vi "FestoCPX.Station.ProdSuctionGripper.SetAll.vi"(8 "error in":errorcluster, 10 "Position":T1) -> (0 "error out":errorcluster)   [LabVIEW 2016]
uses:
  Station/Station.ValvePosition.ctl
  FestoCPX.DO.Signal.ctl
  Station/Station.ProductSuctionGripper.Type.ctl
  FestoCPX.DO.Data.States.Set.vi
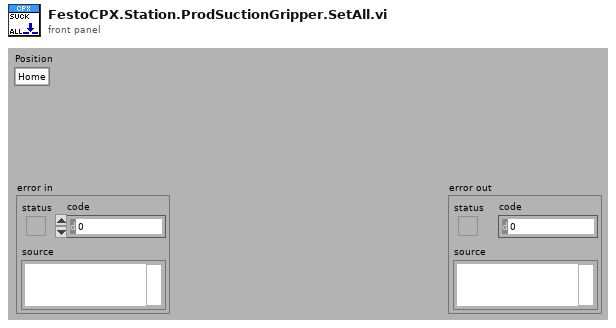
[diagram p1: front panel]
types:
  T1 = typedef "Station.ValvePosition.ctl" = enum16{"Home", "Work"}
  T2 = typedef "FestoCPX.DO.Signal.ctl" = enum16{"Safety Reset", "Air Main Valve", "Door Lock", "Button LED Start", "Button LED Stop", "Button LED Control", "Traffic LED Red", "Traffic LED Orange", "Traffic LED Green", "Horn", "Laser Interlock", "Laser Trigger", "Laser Fume Extractor", "Product Suction Gripper Slot 1 A", "Product Suction Gripper Slot 1 B", "Product Suction Gripper Slot 2 A", "Product Suction Gripper Slot 2 B", "Product Suction Gripper Slot 3 A", "Product Suction Gripper Slot 3 B", "Product Suction Gripper Slot 4 A", "Product Suction Gripper Slot 4 B", "Product Suction Gripper Final A", "Product Suction Gripper Final B", "Lamp", "Q1 Product Move Work", "Q1 Product Move Home", "Q2 Table Turn Work", "Q2 Table Turn Home", "Q3 Product Lift A", "Q3 Product Lift B", "Q4 Product Arm OK", "Q4 Product Arm NOK", "Q5 Product Arm Work", "Q6 Product BlowOut A", "Q6 Product BlowOut B"}
  T3 = typedef "Station.ProductSuctionGripper.Type.ctl" = enum8{"Final A", "Final B", "Slot 1 A", "Slot 1 B", "Slot 2 A", "Slot 2 B", "Slot 3 A", "Slot 3 B", "Slot 4 A", "Slot 4 B"}
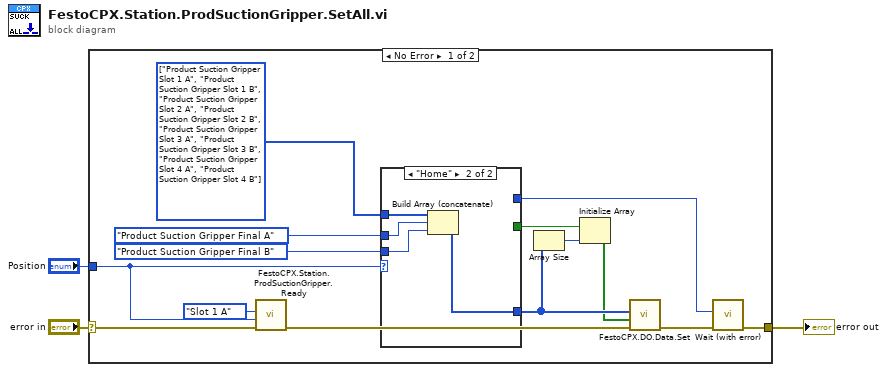
[diagram p0: block diagram]
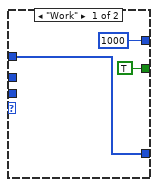
[diagram p2: hidden frame]
diagram:
  n1 = case shown="No Error" "error in" {
    selector: "error in" -> [w16 w25]
    tunnel: [w5 w25] -> w3
    tunnel: "Position" -> [w13 _]
    frame No Error {
      w10 = T2[] [enum."Product Suction Gripper Slot 1 A", enum."Product Suction Gripper Slot 1 B", enum."Product Suction Gripper Slot 2 A", enum."Product Suction Gripper Slot 2 B", enum."Product Suction Gripper Slot 3 A", enum."Product Suction Gripper Slot 3 B", enum."Product Suction Gripper Slot 4 A", enum."Product Suction Gripper Slot 4 B"] items=["Safety Reset", "Air Main Valve", "Door Lock", "Button LED Start", "Button LED Stop", "Button LED Control", "Traffic LED Red", "Traffic LED Orange", "Traffic LED Green", "Horn", "Laser Interlock", "Laser Trigger", "Laser Fume Extractor", "Product Suction Gripper Slot 1 A", "Product Suction Gripper Slot 1 B", "Product Suction Gripper Slot 2 A", "Product Suction Gripper Slot 2 B", "Product Suction Gripper Slot 3 A", "Product Suction Gripper Slot 3 B", "Product Suction Gripper Slot 4 A", "Product Suction Gripper Slot 4 B", "Product Suction Gripper Final A", "Product Suction Gripper Final B", "Lamp", "Q1 Product Move Work", "Q1 Product Move Home", "Q2 Table Turn Work", "Q2 Table Turn Home", "Q3 Product Lift A", "Q3 Product Lift B", "Q4 Product Arm OK", "Q4 Product Arm NOK", "Q5 Product Arm Work", "Q6 Product BlowOut A", "Q6 Product BlowOut B"] ("CPX.DO")
      n2 = call "FestoCPX.Station.ProdSuctionGripper.Ready.vi"("error in"=w16, "Position"=w13, "Type"=Station.ProductSuctionGripper.Type."Slot 1 A") -> ("error out"=w15:errorcluster)  [unwired: 7 in, 1 out]
      n3 = case shown="\"Home\"" w13 {
        tunnel: w10 -> [w20 w24]
        tunnel: FestoCPX.DO.Signal."Product Suction Gripper Final A" ("CPX.DO") -> [_ w23]
        tunnel: FestoCPX.DO.Signal."Product Suction Gripper Final B" ("CPX.DO") -> [_ w22]
        tunnel: [w20 w21] -> w9
        tunnel: [TRUE _] -> w7
        tunnel: [u32 1000 ("milliseconds to wait") _] -> w4
        frame "Work" {
        }
        frame "Home" {
          n4 = Build Array (concatenate)(w24, w23, w22) -> (w21:T2[])
        }
      }
      n5 = Array Size(array=w9) -> (size(s)=w8:i32)
      n6 = Initialize Array(w7, w8) -> (w6:bool[])
      n7 = call-poly "FestoCPX.DO.Data.Set.vi"("error in (no error)"=w15, "State"=w6, "CPX.DO"=w9) -> ("error out"=w17:errorcluster)  [unwired: 8 in]
      n8 = call "Wait (with error).vi"("error in (no error)"=w17, "milliseconds to wait"=w4) -> ("error out"=w5:errorcluster)  [unwired: 8 in, 1 out]
    }
    frame Error {
    }
  }
  "error out" <- w3
